vi "NI VeriStand - Set Channel 2D Array Values.vi"(8 "error in (no error)":errorcluster, 9 "Values":dbl[][](array[numeric]), 10 "Channel":string, 11 "WorkspaceManager in":T1) -> (0 "error out":errorcluster, 3 "WorkspaceManager out":T1)   [LabVIEW 2020, in "NI_VS Workspace ExecutionAPI.lvlib"]
doc: "Sets values of channels on the target. You must manually select the polymorphic instance to use."
uses:
  <vilib>/NI VeriStand/Execution/Workspace/NI_VS Workspace ExecutionAPI.lvlib
  <vilib>/NI VeriStand/Execution/Workspace/WorkspaceAPI.ctl
  NationalInstruments.VeriStand.ClientAPI
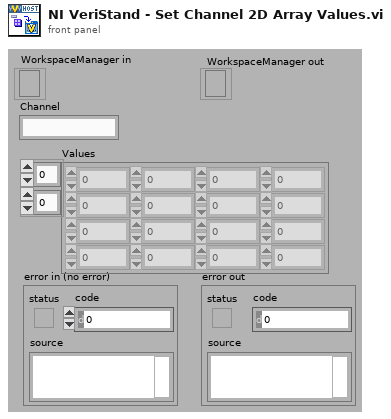
[diagram p1: front panel]
types:
  T1 = typedef "NI_VS Workspace ExecutionAPI.lvlib/WorkspaceAPI.ctl" = refnum<k24>
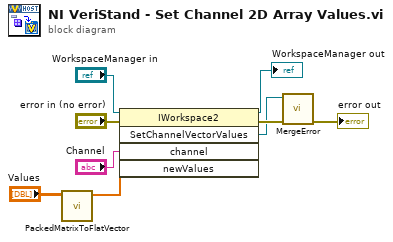
[diagram p0: block diagram]
diagram:
  n1 = call <vilib>:"PackedMatrixToFlatVector.vi"("Matrix"="Values") -> ("FlatVector"=w2:dbl[])  [unwired: 10 out]
  n2 = invoke class="IWorkspace2" method="SetChannelVectorValues"(reference="WorkspaceManager in", error in="error in (no error)", "channel"="Channel", "newValues"=w2) -> (reference out=→"WorkspaceManager out":T1, error out=w7:errorcluster, "SetChannelVectorValues"=w6:refnum<k24>)  [unwired: 1 in, 2 out]
  n3 = call <vilib>:"MergeError.vi"("error in (no error)"=w7, "Error"=w6) -> ("error out"=→"error out":errorcluster)  [unwired: 9 out]
